vi "读取输入输出状态.vi"(8 "error in (no error)":errorcluster, 10 "quantity":u16, 11 "starting address":u16) -> (0 "error out":errorcluster, 3 "Coils":bool[](array[boolean]))   [LabVIEW 2016, in "一代CodMn.lvlib"]
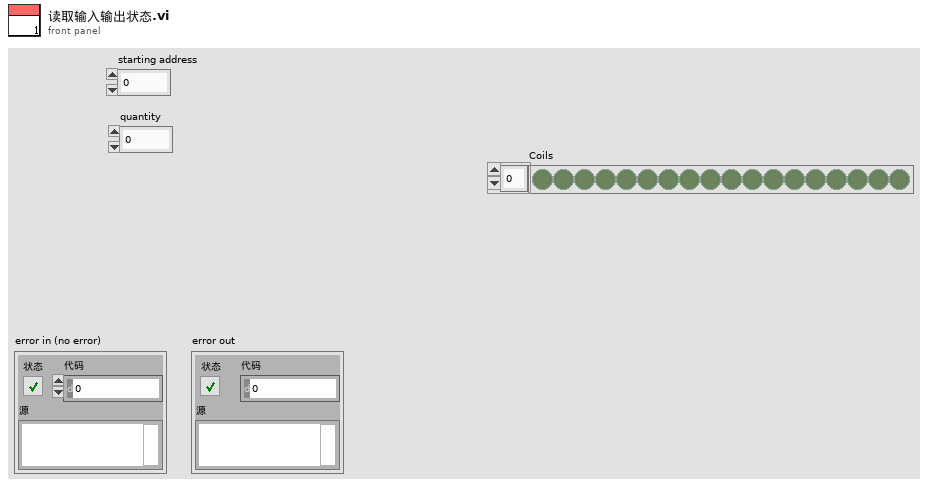
[diagram p1: front panel]
types:
  T1 = enum16{"open", "close", "readHR", "writeHR", "readCoil", "writeCoil"}
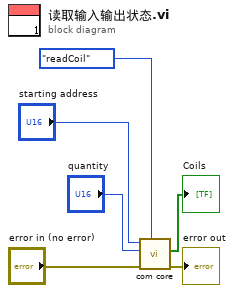
[diagram p0: block diagram]
diagram:
  n1 = call "com core.vi"("功能"=T1."readCoil", "error in (no error)"="error in (no error)", "quantity"="quantity", "starting address"="starting address") -> ("error out"=→"error out":errorcluster, "Coils"=→"Coils":bool[])  [unwired: 5 in, 1 out]
